vi "Find Resources.vi"(3 "error in (no error)":errorcluster {"code" format="%.0x"}) -> (0 "error out":errorcluster, 1 "Resource Names":string[](array[string]), 2 "Count":u32 caption="Resource Count")   [LabVIEW 2017, in "OPM.ThorlabsPM400.lvclass"]
uses:
  OPM.ThorlabsPM400.lvclass
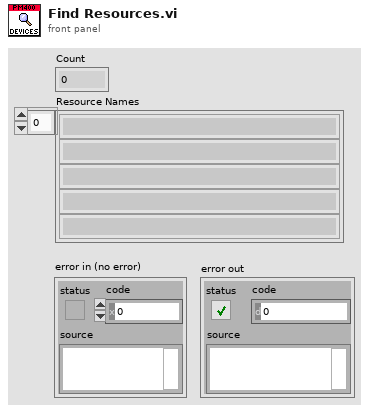
[diagram p1: front panel]
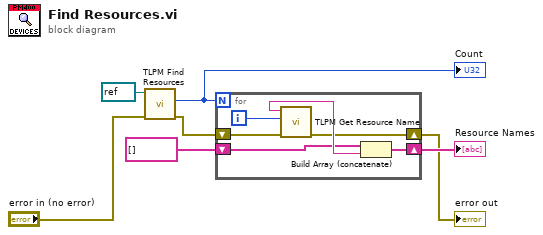
[diagram p0: block diagram]
diagram:
  n1 = call <instrlib>:"TLPM Find Resources.vi"("error in (no error)"="error in (no error)", "instrument handle"=refnum<visa-resource-name> refnum) -> ("error out"=w2:errorcluster, "Resource Count"=w6:u32)  [unwired: 7 in, 1 out]
  "Count" <- w6
  n2 = for {
    N: w6 -> [_]
    shift-right: [w11] -> w5
    shift-left: string[] [] ("appended array") -> [w10]
    shift-right: [w8] -> w1
    shift-left: w2 -> [w9]
    i -> [w13]
    n3 = call <instrlib>:"TLPM Get Resource Name.vi"("error in (no error)"=w9, "Index (0)"=w13) -> ("error out"=w8:errorcluster, "Resource Name"=w12:string)  [unwired: 7 in, 1 out]
    n4 = Build Array (concatenate)(w10, w12) -> (w11:string[])
  }
  "Resource Names" <- w5
  "error out" <- w1
